vi "2D String To 1D I64.vi"(10 "2D String In":string[][](array[string])) -> (2 "1D I64":i64[](array[numeric]))   [LabVIEW 2024]
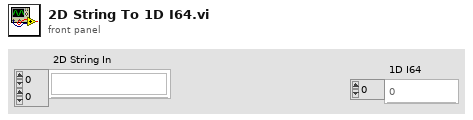
[diagram p1: front panel]
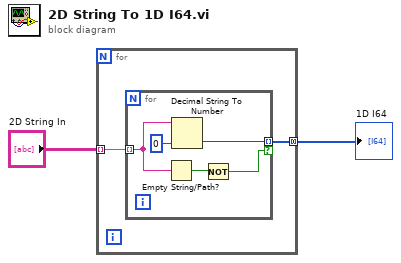
[diagram p0: block diagram]
diagram:
  n1 = for {
    tunnel: "2D String In" -> [w4] mode=indexing
    tunnel: [w3] -> w1 mode=concatenating
    n2 = for {
      tunnel: w4 -> [w9] mode=indexing
      tunnel: [w7] -> w3 mode=indexing if=w6
      n3 = Empty String/Path?(string/path=w9) -> (empty?=w8:bool)
      n4 = Decimal String To Number(string=w9, default (0L)=i64 0 ("default (0 I32)")) -> (number=w7:i64)  [unwired: 1 in, 1 out]
      n5 = Not(x=w8) -> (.not. x?=w6:bool)
    }
  }
  "1D I64" <- w1
